vi "RT_Main.vi"() -> ()   [LabVIEW 2019]
uses:
  <vilib>/Instr/_visa.llb/VISA Configure Serial Port (Serial Instr).vi
panel:
  in  "E-Shutdown":bool
  out "Process Errors":errorcluster
  in  "Log Drycal":bool=TRUE
  out "Running?":bool
  out "Shutdown Activated?":bool
  out "Alicat Errors":errorcluster
  # "Bypass Drycal"
  # "Starting this code:\nStep 1:\n- Open transducers to atmopheric \n   pressure\nStep 2:\n- Start program\nStep 3:\n- Close transducers\nStep 4:\n- Continue normal operation"
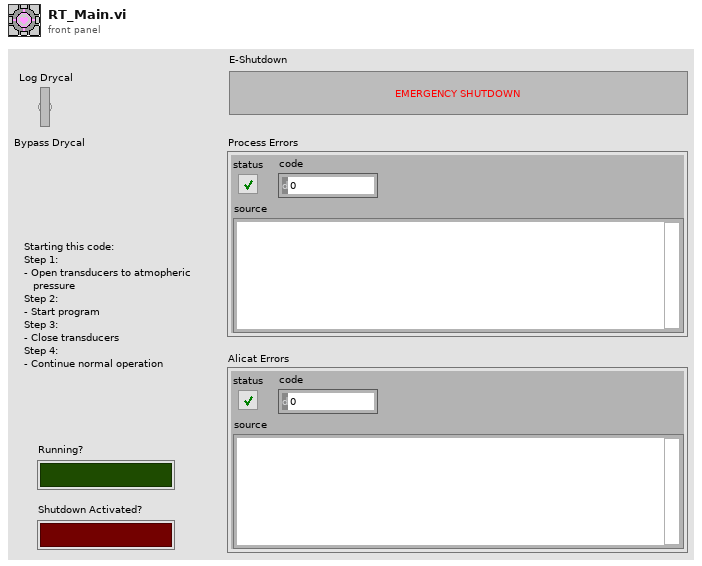
[diagram p1: front panel]
types:
  T1 = cluster{"Unit ID":string, "Baud Rate":enum8{"2400", "9600", "19200", "38400", "57600", "115200", "Unknown"}, "VISA Sesssion In":refnum<visa-resource-name>}
  T2 = cluster{"Array of String":string[], "Array of Double":dbl[], "Array of Double":dbl[]}
  T3 = cluster{"Array of String":string[], dbl[], "Array of Double":dbl[]}
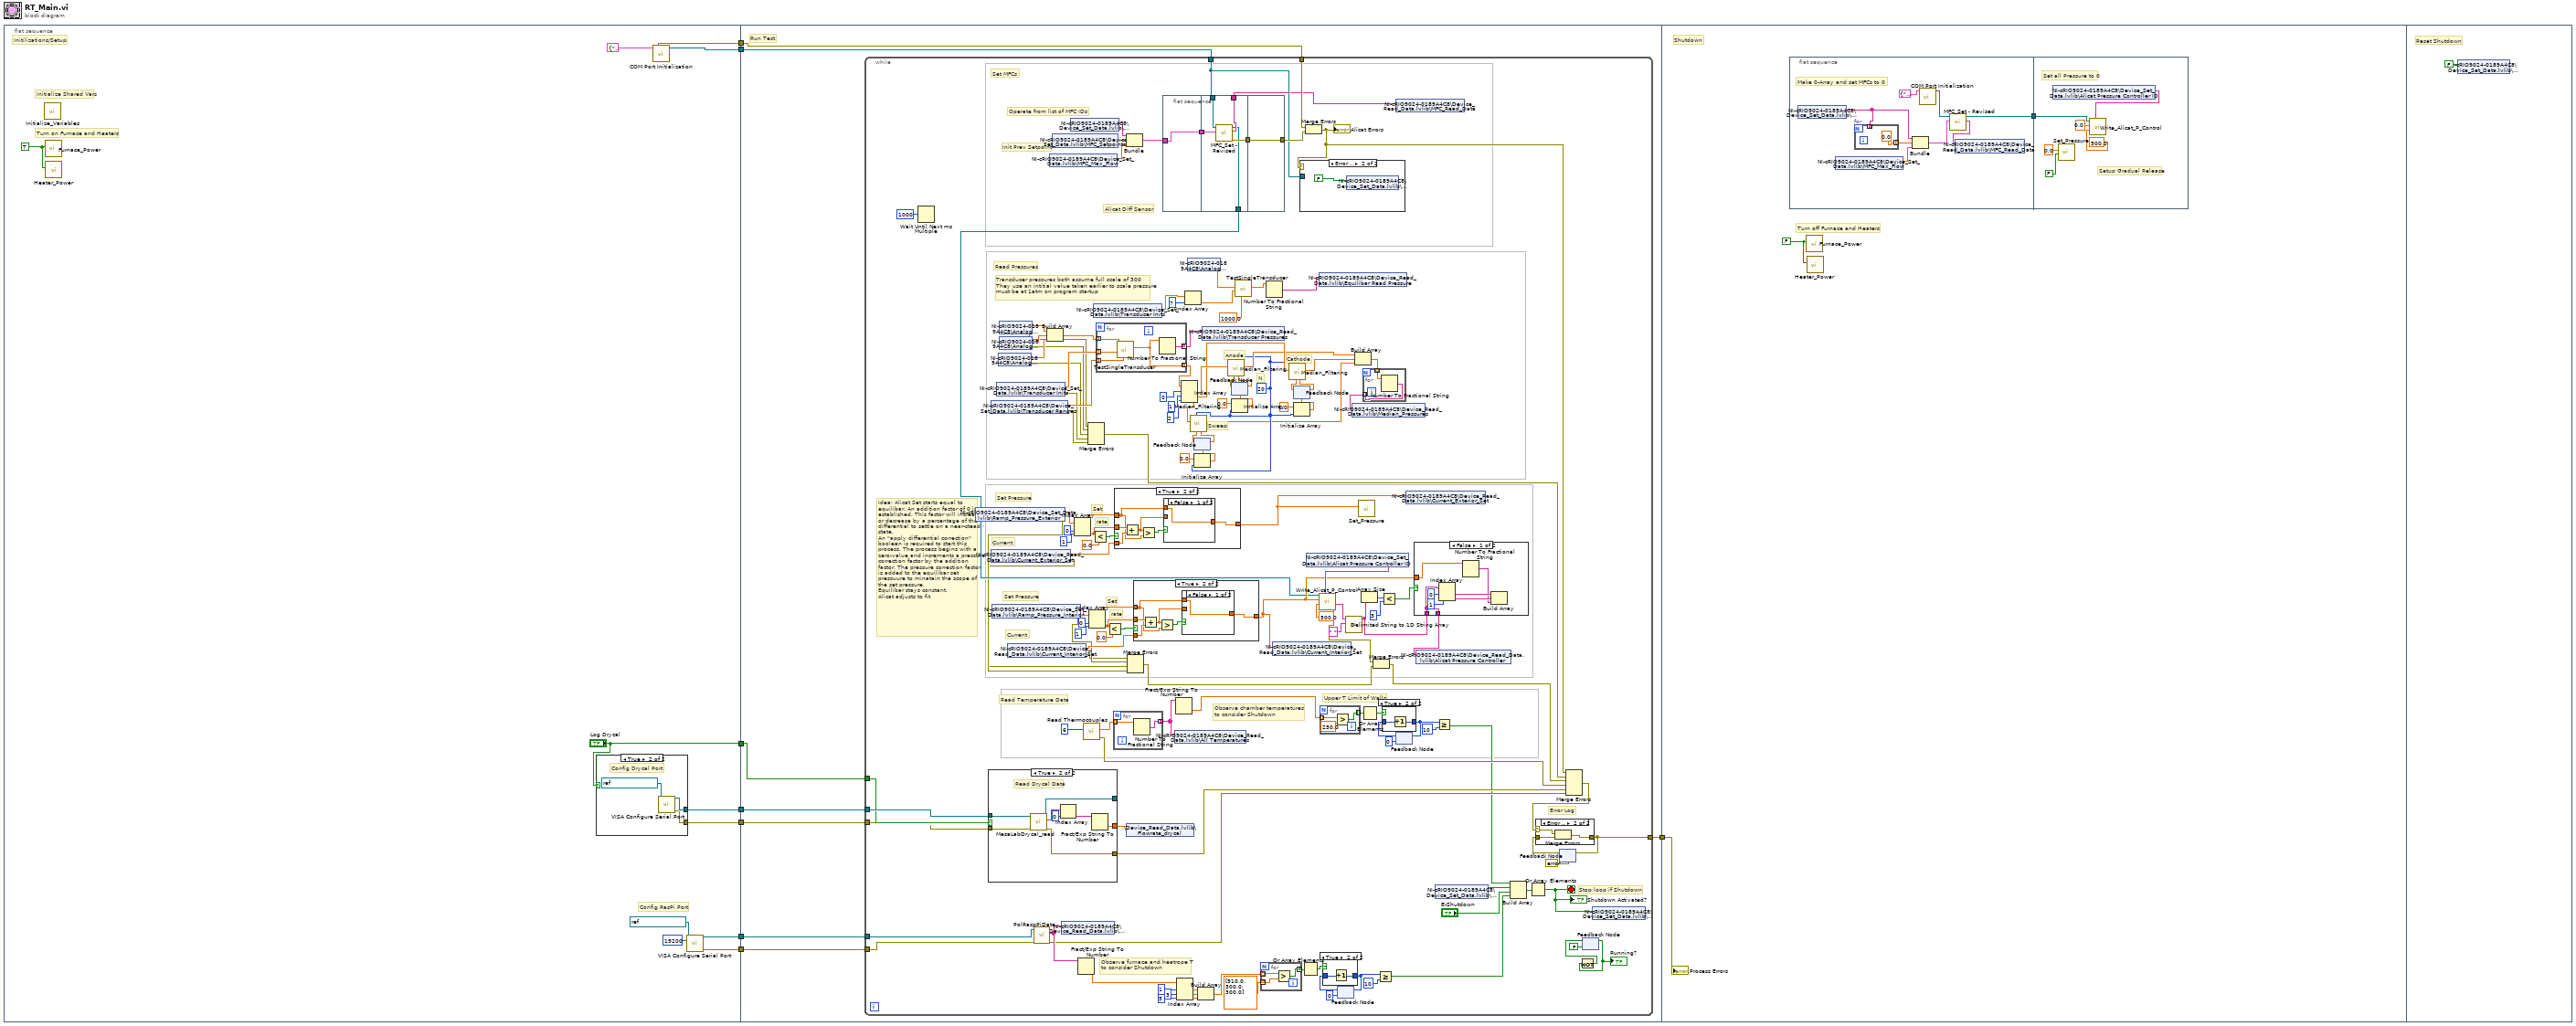
[diagram p0: block diagram]
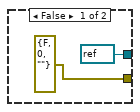
[diagram p2: hidden frame]
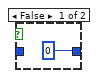
[diagram p3: hidden frame]
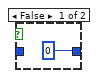
[diagram p4: hidden frame]
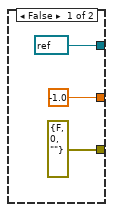
[diagram p6: hidden frame]
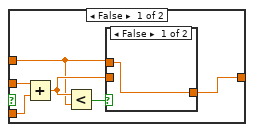
[diagram p7: hidden frame]
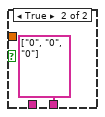
[diagram p10: hidden frame]
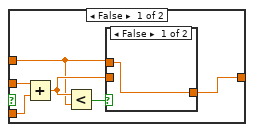
[diagram p11: hidden frame]
diagram:
  n1 = flat-sequence {
    tunnel: [w19] -> w8
    tunnel: [w18] -> w7
    tunnel: [w16] -> w6
    tunnel: ["Log Drycal"] -> w5
    tunnel: [w14] -> w4
    tunnel: [w12] -> w3
    tunnel: [w11] -> w2
    tunnel: w8 -> [w32]
    tunnel: w7 -> [w31]
    tunnel: w6 -> [w30]
    tunnel: w5 -> [w29]
    tunnel: w4 -> [w28]
    tunnel: w3 -> [w27]
    tunnel: w2 -> [w26]
    tunnel: [w25] -> w1
    tunnel: w1 -> [w258]
    frame #0 {
      w9 = TRUE ("Furnace Power (off)")
      # "Turn on Furnace and Heaters"
      # "Config RasPi Port"
      # "Initialize Shared Vars"
      # "Initilizations/Setup"
      n2 = call "Initialize_Variables.vi"() -> ()  [unwired: 12 in]
      n3 = call "Furnace_Power.vi"("Furnace Power (off)"=w9) -> ()  [unwired: 10 in, 1 out]
      n4 = call "Heater_Power.vi"("Furnace Power (off)"=w9) -> ()  [unwired: 10 in, 1 out]
      n5 = case shown="True" "Log Drycal" {
        tunnel: [refnum<visa-resource-name> refnum ("VISA resource name out") w23] -> w16
        tunnel: [errorcluster {"status"=FALSE, "code"=0, "source"=""} ("error out") w22] -> w14
        frame False {
        }
        frame True {
          # "Config Drycal Port"
          n6 = call-poly "VISA Configure Serial Port"("VISA resource name"=refnum<visa-resource-name> "ASRL11::INSTR" ("VISA Sesssion In")) -> ("VISA resource name out"=w23:refnum<visa-resource-name>, "error out"=w22:errorcluster)  [unwired: 13 in]
        }
      }
      n7 = call <instrlib>:"COM Port Initialization.vi"("Communication Settings"=T1 {"Unit ID"="A", "Baud Rate"=enum."19200", "VISA Sesssion In"="ASRL13::INSTR"}) -> ("error out"=w19:errorcluster, "VISA Session Out"=w18:refnum<visa-resource-name>)  [unwired: 9 in]
      n8 = call-poly "VISA Configure Serial Port"("VISA resource name"=refnum<visa-resource-name> "ASRL12::INSTR" ("VISA Sesssion In"), "baud rate (9600)"=u32 19200) -> ("VISA resource name out"=w11:refnum<visa-resource-name>, "error out"=w12:errorcluster)  [unwired: 12 in]
    }
    frame #1 {
      # "Run Test"
      n9 = while {
        tunnel: w32 -> [w153]
        tunnel: w31 -> [w152]
        tunnel: w30 -> [w98]
        tunnel: w29 -> [w97]
        tunnel: w28 -> [w95]
        tunnel: w26 -> [w94]
        tunnel: w27 -> [w93]
        tunnel: [w60] -> w25
        stop <- w38 stop-if-true
        w85 = 20 ("N")
        # "Set MFCs"
        # "Upper T Limit of Walls"
        # "Error Log"
        # "Observe chamber temperatures \nto consider Shutdown"
        # "Observe furnace and heatrope T\nto consider Shutdown"
        # "Sweep"
        # "N"
        # "Cathode"
        # "Current"
        # "rate"
        # "Set"
        # "Set Pressure"
        # "Anode"
        # "Idea: Alicat Set starts equal to equilibar. An addition factor of 0 is established. This factor will increase or decrease by a percentage of the differential to settle on a near-steady state.\nAn \"apply differential correction\" boolean is required to start this process. The process begins with a zero-value and increments a pressure correction factor by the addition factor. The pressure correction factor is added to the equilibar set pressuure to minatain the scope of the set pressure.\nEquilibar stays constant,\nAlicat adjusts to fit"
        # "Transducer pressures both assume full scale of 300\nThey use an intitial value taken earlier to scale pressure\nmust be at 1atm on program startup"
        # "Read Temperature Data"
        # "Alicat Diff Sensor"
        # "Read Pressures"
        # "Current"
        # "rate"
        # "Set"
        # "Set Pressure"
        # "Stop loop if Shutdown"
        # "Operate from list of MFC IDs"
        # "Init Prev Setpoint"
        n10 = Wait Until Next ms Multiple(millisecond multiple=u32 1000) -> ()  [unwired: 1 out]
        n11 = shared-variable "NI-cRIO9024-0189A4C8\\Device_Set_Data.lvlib\\Ramp_Pressure_Exterior"() -> (w165:dbl[], error out=w70:errorcluster)  [unwired: 1 in]
        n12 = case shown="True" w97 {
          tunnel: w98 -> [_ w199]
          tunnel: [-1.0 w198] -> w96
          tunnel: w95 -> [_ w197]
          tunnel: [refnum<visa-resource-name> refnum ("VISA Sesssion Out") w193] -> _
          tunnel: [errorcluster {"status"=FALSE, "code"=0, "source"=""} ("error out") w192] -> w62
          frame False {
          }
          frame True {
            # "Read Drycal Data"
            n13 = call "MesaLabDrycal_read.vi"("error in (no error)"=w197, "VISA Sesssion In"=w199) -> ("error out"=w192:errorcluster, "output array"=w196:string[], "VISA Sesssion Out"=w193:refnum<visa-resource-name>)  [unwired: 7 in]
            n14 = Index Array(array=w196, index=0) -> (element=w194:string)
            n15 = Fract/Exp String To Number(string=w194) -> (number=w198:dbl)  [unwired: 3 in, 1 out]
          }
        }
        n16 = shared-variable "NI-cRIO9024-0189A4C8\\Device_Read_Data.lvlib\\Current_Exterior_Set"() -> (w151:dbl, error out=w69:errorcluster)  [unwired: 1 in]
        n17 = shared-variable "NI-cRIO9024-0189A4C8\\Device_Set_Data.lvlib\\Transducer Ranges"() -> (w146:dbl[], error out=w72:errorcluster)  [unwired: 1 in]
        n18 = shared-variable "NI-cRIO9024-0189A4C8\\Device_Set_Data.lvlib\\Ramp_Pressure_Interior"() -> (w121:dbl[], error out=w68:errorcluster)  [unwired: 1 in]
        n19 = shared-variable "NI-cRIO9024-0189A4C8\\Device_Set_Data.lvlib\\Transducer Inits"() -> (w148:dbl[], error out=w73:errorcluster)  [unwired: 1 in]
        n20 = shared-variable "NI-cRIO9024-0189A4C8\\Analog Current In\\AI2"() -> (w92:dbl, error out=w74:errorcluster)  [unwired: 1 in]
        n21 = shared-variable "NI-cRIO9024-0189A4C8\\Analog Current In\\AI0"() -> (w150:dbl, error out=w76:errorcluster)  [unwired: 1 in]
        n22 = shared-variable "NI-cRIO9024-0189A4C8\\Analog Current In\\AI1"() -> (w149:dbl, error out=w75:errorcluster)  [unwired: 1 in]
        n23 = shared-variable "NI-cRIO9024-0189A4C8\\Device_Read_Data.lvlib\\Current_Interior_Set"() -> (w122:dbl, error out=w67:errorcluster)  [unwired: 1 in]
        n24 = call "PolRaspPiData.vi"("error in (no error)"=w93, "VISA Sesssion In"=w94) -> ("error out"=w61:errorcluster, "output array"=w83:string[])  [unwired: 7 in, 1 out]
        n25 = Build Array(w150, w149, w92) -> (w147:dbl[])
        n26 = shared-variable "NI-cRIO9024-0189A4C8\\Device_Set_Data.lvlib\\MFC_Max_Flow"() -> (w170:dbl[])  [unwired: 1 in, 1 out]
        n27 = shared-variable "NI-cRIO9024-0189A4C8\\Device_Set_Data.lvlib\\MFC_Setpoints"() -> (w171:dbl[])  [unwired: 1 in, 1 out]
        n28 = shared-variable "NI-cRIO9024-0189A4C8\\Device_Read_Data.lvlib\\Raspi Data"(w83) -> ()  [unwired: 1 in, 1 out]
        n29 = shared-variable "NI-cRIO9024-0189A4C8\\Device_Set_Data.lvlib\\MFC_IDs"() -> (w172:string[])  [unwired: 1 in, 1 out]
        n30 = Index Array(array=w165, index #1=0 ("index"), index #2=1 ("index")) -> (element #1=w159:dbl, element #2=w160:dbl)
        n31 = Fract/Exp String To Number(string=w83) -> (number=w82:dbl[])  [unwired: 3 in, 1 out]
        n32 = call "Read Thermocouples.vi"("Thermocouple Count (15)"=6) -> ("error out"=w63:errorcluster, "Temperatures (C)"=w154:dbl[])  [unwired: 9 in]
        n33 = Merge Errors(w76, w75, w74, w73, w72) -> (w71:errorcluster)
        n34 = Index Array(array=w121, index #1=0 ("index"), index #2=1 ("index")) -> (element #1=w123:dbl, element #2=w124:dbl)
        n35 = Less?(x=w160, y=0.0) -> (x < y?=w161:bool)
        n36 = shared-variable "NI-cRIO9024-0189A4C8\\Device_Set_Data.lvlib\\Transducer Inits"() -> (w118:dbl[])  [unwired: 1 in, 1 out]
        n37 = for {
          tunnel: w148 -> [w230] mode=indexing
          tunnel: w147 -> [w229] mode=indexing
          tunnel: w146 -> [w228] mode=indexing
          tunnel: [w227] -> w141 mode=indexing
          tunnel: [w226] -> w104 mode=indexing
          n38 = call "TestSingleTransducer.vi"("Full Range"=w228, "Reference"=w230, "Analog In"=w229) -> ("Pressure"=w227:dbl)  [unwired: 8 in]
          n39 = Number To Fractional String(number=w227) -> (F-format string=w226:string)  [unwired: 3 in]
        }
        n40 = Less?(x=w124, y=0.0) -> (x < y?=w125:bool)
        n41 = for {
          tunnel: w154 -> [w232] mode=indexing
          tunnel: [w231] -> w81 mode=indexing
          n42 = Number To Fractional String(number=w232) -> (F-format string=w231:string)  [unwired: 3 in]
        }
        n43 = case shown="True" w161 {
          tunnel: w159 -> [w240 w248]
          tunnel: w160 -> [w245 w253]
          tunnel: w151 -> [w244 w252]
          tunnel: [w241 w249] -> w129
          frame False {
            n44 = Add(x=w245, y=w244) -> (x+y=w242:dbl)
            n45 = Less?(x=w242, y=w240) -> (x < y?=w243:bool)
            n46 = case shown="False" w243 {
              tunnel: w242 -> [_ w247]
              tunnel: [w246 w247] -> w241
              tunnel: w240 -> [w246 _]
              frame False {
              }
              frame True {
              }
            }
          }
          frame True {
            n47 = Add(x=w253, y=w252) -> (x+y=w250:dbl)
            n48 = Greater?(x=w250, y=w248) -> (0:w251:bool)
            n49 = case shown="False" w251 {
              tunnel: w250 -> [_ w255]
              tunnel: [w254 w255] -> w249
              tunnel: w248 -> [w254 _]
              frame False {
              }
              frame True {
              }
            }
          }
        }
        n50 = Bundle("Array of String"=w172, "Array of Double"=w171, "Array of Double"=w170) -> (w169:T2)  [unwired: 1 in]
        n51 = shared-variable ".\\Device_Read_Data.lvlib\\Flowrate_drycal"(w96) -> ()  [unwired: 1 in, 1 out]
        n52 = Merge Errors(w67, w68, w69, w70) -> (w65:errorcluster)
        n53 = case shown="True" w125 {
          tunnel: w123 -> [w202 w210]
          tunnel: w124 -> [w207 w215]
          tunnel: w122 -> [w206 w214]
          tunnel: [w203 w211] -> w120
          frame False {
            n54 = Add(x=w207, y=w206) -> (x+y=w204:dbl)
            n55 = Less?(x=w204, y=w202) -> (x < y?=w205:bool)
            n56 = case shown="False" w205 {
              tunnel: w204 -> [_ w209]
              tunnel: [w208 w209] -> w203
              tunnel: w202 -> [w208 _]
              frame False {
              }
              frame True {
              }
            }
          }
          frame True {
            n57 = Add(x=w215, y=w214) -> (x+y=w212:dbl)
            n58 = Greater?(x=w212, y=w210) -> (0:w213:bool)
            n59 = case shown="False" w213 {
              tunnel: w212 -> [_ w217]
              tunnel: [w216 w217] -> w211
              tunnel: w210 -> [w216 _]
              frame False {
              }
              frame True {
              }
            }
          }
        }
        n60 = flat-sequence {
          tunnel: w169 -> [w233]
          tunnel: [w233] -> w157
          tunnel: [w237] -> w158
          tunnel: w157 -> [w238]
          tunnel: [w236] -> w116
          tunnel: w152 -> [w235]
          tunnel: [w234] -> w100
          tunnel: [w239] -> w156
          tunnel: w158 -> [w239]
          frame #0 {
          }
          frame #1 {
            n61 = call "MFC_Set - Revised.vi"("MFC info"=w238, "VISA Session In"=w235) -> ("error out"=w237:errorcluster, "MFC_Data"=w236:string[], "VISA Sesssion Out"=w234:refnum<visa-resource-name>)  [unwired: 7 in]
          }
          frame #2 {
          }
        }
        n62 = shared-variable "NI-cRIO9024-0189A4C8\\Device_Read_Data.lvlib\\All Temperatures"(w81) -> ()  [unwired: 1 in, 1 out]
        n63 = Fract/Exp String To Number(string=w81) -> (number=w59:dbl[])  [unwired: 3 in, 1 out]
        n64 = Index Array(array=w82, index #1=1 ("index"), index #2=3 ("index"), index #3=5 ("index")) -> (element #1=w45:dbl, element #2=w43:dbl, element #3=w44:dbl)
        n65 = Index Array(array=w141, index #1=0 ("index"), index #2=1 ("index"), index #3=2 ("index")) -> (element #1=w111:dbl, element #2=w106:dbl, element #3=w86:dbl)
        n66 = Index Array(array=w118, index=7) -> (element=w117:dbl)
        n67 = shared-variable "NI-cRIO9024-0189A4C8\\Analog Current In\\AI7"() -> (w139:dbl)  [unwired: 1 in, 1 out]
        n68 = Initialize Array(0.0 ("element"), w85) -> (w88:dbl[])
        n69 = feedback #1(w88) -> (w90:dbl[])
        n70 = call "Median_Filtering.vi"("Feedback Array"=w90, "N"=w85, "CurrentValue"=w86) -> ("Median Value"=w84:dbl, "Array to Back Feed"=w91:dbl[])  [unwired: 7 in]
        n71 = feedback-in #1(w91) -> ()
        n72 = Build Array(w45, w43, w44) -> (w40:dbl[])
        n73 = shared-variable "NI-cRIO9024-0189A4C8\\Device_Read_Data.lvlib\\Transducer Pressures"(w104) -> ()  [unwired: 1 in, 1 out]
        n74 = Initialize Array(0.0 ("element"), w85) -> (w112:dbl[])
        n75 = feedback #2(w112) -> (w114:dbl[])
        n76 = call "Median_Filtering.vi"("Feedback Array"=w114, "N"=w85, "CurrentValue"=w111) -> ("Median Value"=w102:dbl, "Array to Back Feed"=w115:dbl[])  [unwired: 7 in]
        n77 = feedback-in #2(w115) -> ()
        n78 = call "TestSingleTransducer.vi"("Full Range"=1000.0, "Reference"=w117, "Analog In"=w139) -> ("Pressure"=w137:dbl)  [unwired: 8 in]
        n79 = for {
          tunnel: w40 -> [w174] mode=indexing
          tunnel: [w175] -> w42 mode=indexing
          tunnel: dbl[] [910.0, 300.0, 300.0] ("appended array") -> [w173] mode=indexing
          n80 = Greater?(x=w174, y=w173) -> (0:w175:bool)
        }
        n81 = Number To Fractional String(number=w137) -> (F-format string=w136:string)  [unwired: 3 in]
        n82 = shared-variable "NI-cRIO9024-0189A4C8\\Device_Read_Data.lvlib\\Current_Interior_Set"(w120) -> ()  [unwired: 1 in, 1 out]
        n83 = Initialize Array(0.0 ("element"), w85) -> (w107:dbl[])
        n84 = feedback #3(w107) -> (w109:dbl[])
        n85 = call "Median_Filtering.vi"("Feedback Array"=w109, "N"=w85, "CurrentValue"=w106) -> ("Median Value"=w101:dbl, "Array to Back Feed"=w110:dbl[])  [unwired: 7 in]
        n86 = feedback-in #3(w110) -> ()
        n87 = Or Array Elements(Boolean array=w42) -> (logical OR=w41:bool)
        n88 = Merge Errors(w153, w156) -> (w77:errorcluster)
        "Alicat Errors" <- w77
        n89 = case shown="Error .." w77 {
          tunnel: w152 -> [_ _]
          frame No Error {
          }
          frame Error {
            n90 = shared-variable "NI-cRIO9024-0189A4C8\\Device_Set_Data.lvlib\\Shutdown"(FALSE ("Shutdown")) -> ()  [unwired: 1 in, 1 out]
          }
        }
        n91 = shared-variable "NI-cRIO9024-0189A4C8\\Device_Set_Data.lvlib\\Alicat Pressure Controller ID"() -> (w144:string)  [unwired: 1 in, 1 out]
        n92 = shared-variable "NI-cRIO9024-0189A4C8\\Device_Read_Data.lvlib\\Equilibar Read Pressure"(w136) -> ()  [unwired: 1 in, 1 out]
        n93 = call "Write_Alicat_P_Control.vi"("Device ID (G)"=w144, "Device Range"=500.0, "Set Point"=w120, "VISA Sesssion In"=w100) -> ("error out"=w66:errorcluster, "read buffer"=w135:string)  [unwired: 4 in, 2 out]
        n94 = for {
          tunnel: w59 -> [w182] mode=indexing
          tunnel: [w183] -> w55 mode=indexing
          n95 = Greater?(x=w182, y=250.0) -> (0:w183:bool)
        }
        n96 = feedback #4(0) -> (w52:i32)
        n97 = case shown="True" w41 {
          tunnel: [0 w178] -> w50
          tunnel: w52 -> [_ w177]
          frame False {
          }
          frame True {
            n98 = Increment(x=w177) -> (x+1=w178:i32)
          }
        }
        n99 = feedback-in #4(w50) -> ()
        n100 = call <vilib>:"Delimited String to 1D String Array.vi"("delimiter"=" ", "delimited string"=w135) -> ("string array"=w131:string[])  [unwired: 9 in]
        n101 = Build Array(w102, w101, w84) -> (w105:dbl[])
        n102 = call "Set_Pressure.vi"("Set Pressure (PSI)"=w129) -> ()  [unwired: 10 in, 1 out]
        n103 = Array Size(array=w131) -> (size(s)=w134:i32)
        n104 = Or Array Elements(Boolean array=w55) -> (logical OR=w56:bool)
        n105 = for {
          tunnel: w105 -> [w201] mode=indexing
          tunnel: [w200] -> w103 mode=indexing
          n106 = Number To Fractional String(number=w201) -> (F-format string=w200:string)  [unwired: 3 in]
        }
        n107 = shared-variable "NI-cRIO9024-0189A4C8\\Device_Read_Data.lvlib\\Median_Pressures"(w103) -> ()  [unwired: 1 in, 1 out]
        n108 = Merge Errors(w66, w65) -> (w64:errorcluster)
        n109 = Greater Or Equal?(x=w50, y=10) -> (x >= y?=w34:bool)
        n110 = Less?(x=w134, y=3) -> (x < y?=w132:bool)
        n111 = shared-variable "NI-cRIO9024-0189A4C8\\Device_Read_Data.lvlib\\MFC_Read_Data"(w116) -> ()  [unwired: 1 in, 1 out]
        n112 = feedback #5(0) -> (w58:i32)
        n113 = case shown="True" w56 {
          tunnel: [0 w181] -> w54
          tunnel: w58 -> [_ w180]
          frame False {
          }
          frame True {
            n114 = Increment(x=w180) -> (x+1=w181:i32)
          }
        }
        n115 = feedback-in #5(w54) -> ()
        n116 = shared-variable "NI-cRIO9024-0189A4C8\\Device_Read_Data.lvlib\\Current_Exterior_Set"(w129) -> ()  [unwired: 1 in, 1 out]
        n117 = case shown="False" w132 {
          tunnel: w131 -> [w222 _]
          tunnel: [w222 string[] ["0", "0", "0"] ("string array")] -> w130
          tunnel: w120 -> [w219 _]
          frame False {
            n118 = Index Array(array=w222, index #1=0 ("index"), index #2=1 ("index")) -> (element #1=w221:string, element #2=w220:string)
            n119 = Number To Fractional String(number=w219) -> (F-format string=w218:string)  [unwired: 3 in]
            n120 = Build Array(w221, w220, w218) -> ()  [unwired: 1 out]
          }
          frame True {
          }
        }
        n121 = shared-variable "NI-cRIO9024-0189A4C8\\Device_Read_Data.lvlib\\Alicat Pressure Controller"(w130) -> ()  [unwired: 1 in, 1 out]
        n122 = shared-variable "NI-cRIO9024-0189A4C8\\Device_Set_Data.lvlib\\Shutdown"() -> (w35:bool)  [unwired: 1 in, 1 out]
        n123 = Greater Or Equal?(x=w54, y=10) -> (x >= y?=w33:bool)
        n124 = Build Array(w33, w35, "E-Shutdown", w34) -> (w36:bool[])
        n125 = Or Array Elements(Boolean array=w36) -> (logical OR=w38:bool)
        "Shutdown Activated?" <- w38
        n126 = feedback #6(errorcluster {"status"=FALSE, "code"=0, "source"=""} ("error out")) -> (w80:errorcluster)
        n127 = Merge Errors(w77, w71, w64, w63, w62, w61) -> (w78:errorcluster)
        n128 = case shown="Error .." w78 {
          selector: w78 -> [_ w187]
          tunnel: w80 -> [w185 w188]
          tunnel: [w185 w186] -> w60
          frame No Error {
          }
          frame Error {
            n129 = Merge Errors(w187, w188) -> (w186:errorcluster)
          }
        }
        n130 = feedback-in #6(w60) -> ()
        n131 = feedback #7(FALSE) -> (w166:bool)
        "Running?" <- w166
        n132 = Not(x=w166) -> (.not. x?=w168:bool)
        n133 = feedback-in #7(w168) -> ()
        n134 = shared-variable "NI-cRIO9024-0189A4C8\\Device_Set_Data.lvlib\\Shutdown"(w38) -> ()  [unwired: 1 in, 1 out]
      }
    }
    frame #2 {
      w257 = FALSE ("Furnace Power (off)")
      # "Turn off Furnace and Heaters"
      # "Shutdown"
      n135 = flat-sequence {
        tunnel: [w260] -> w259
        tunnel: w259 -> [w269]
        frame #0 {
          # "Make 0-Array and set MFCs to 0"
          n136 = shared-variable "NI-cRIO9024-0189A4C8\\Device_Set_Data.lvlib\\MFC_IDs"() -> (w264:string[])  [unwired: 1 in, 1 out]
          n137 = shared-variable "NI-cRIO9024-0189A4C8\\Device_Set_Data.lvlib\\MFC_Max_Flow"() -> (w267:dbl[])  [unwired: 1 in, 1 out]
          n138 = for {
            tunnel: w264 -> [_] mode=indexing
            tunnel: [0.0] -> w263 mode=indexing
          }
          n139 = Bundle("Array of String"=w264, w263, "Array of Double"=w267) -> (w266:T3)  [unwired: 1 in]
          n140 = call <instrlib>:"COM Port Initialization.vi"("Communication Settings"=T1 {"Unit ID"="A", "Baud Rate"=enum."19200", "VISA Sesssion In"="ASRL13::INSTR"}) -> ("VISA Session Out"=w261:refnum<visa-resource-name>)  [unwired: 9 in, 1 out]
          n141 = call "MFC_Set - Revised.vi"("MFC info"=w266, "VISA Session In"=w261) -> ("MFC_Data"=w265:string[], "VISA Sesssion Out"=w260:refnum<visa-resource-name>)  [unwired: 7 in, 1 out]
          n142 = shared-variable "NI-cRIO9024-0189A4C8\\Device_Read_Data.lvlib\\MFC_Read_Data"(w265) -> ()  [unwired: 1 in, 1 out]
        }
        frame #1 {
          # "Setup Gradual Release"
          # "Set all Pressure to 0"
          n143 = shared-variable "NI-cRIO9024-0189A4C8\\Device_Set_Data.lvlib\\Alicat Pressure Controller ID"() -> (w274:string)  [unwired: 1 in, 1 out]
          n144 = call "Set_Pressure.vi"("Current Out Mode"=FALSE, "Set Pressure (PSI)"=0.0) -> ()  [unwired: 9 in, 1 out]
          n145 = call "Write_Alicat_P_Control.vi"("Device ID (G)"=w274, "Device Range"=500.0, "Set Point"=0.0, "VISA Sesssion In"=w269) -> ()  [unwired: 4 in, 4 out]
        }
      }
      n146 = call "Furnace_Power.vi"("Furnace Power (off)"=w257) -> ()  [unwired: 10 in, 1 out]
      n147 = call "Heater_Power.vi"("Furnace Power (off)"=w257) -> ()  [unwired: 10 in, 1 out]
      "Process Errors" <- w258
    }
    frame #3 {
      # "Reset Shutdown"
      n148 = shared-variable "NI-cRIO9024-0189A4C8\\Device_Set_Data.lvlib\\Shutdown"(FALSE ("Shutdown")) -> ()  [unwired: 1 in, 1 out]
    }
  }
